vi "TCP - Asynchronous Read of One JSON Message.vi"(8 "error in":errorcluster, 11 "TCP Network Connection in":refnum<k5>) -> (0 "error out":errorcluster, 2 "Received JSON Message":string, 3 "TCP Network Connection out":refnum<k5>)   [LabVIEW 2021]
doc: "Receive a JSON messsage through TCP"
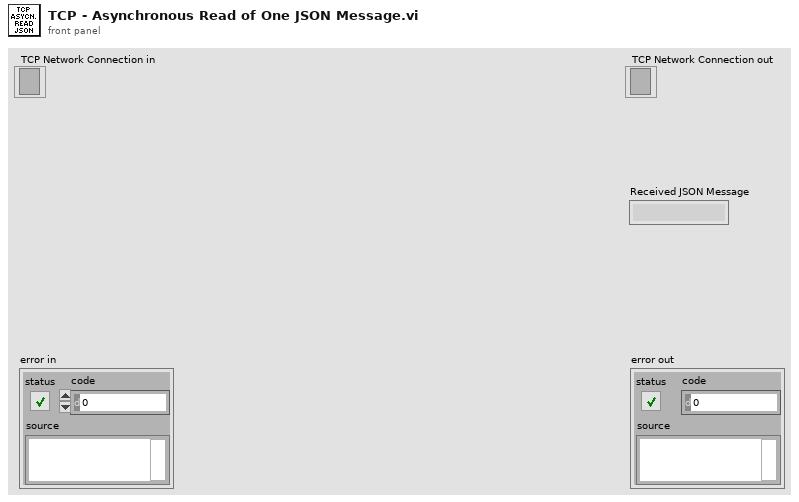
[diagram p1: front panel]
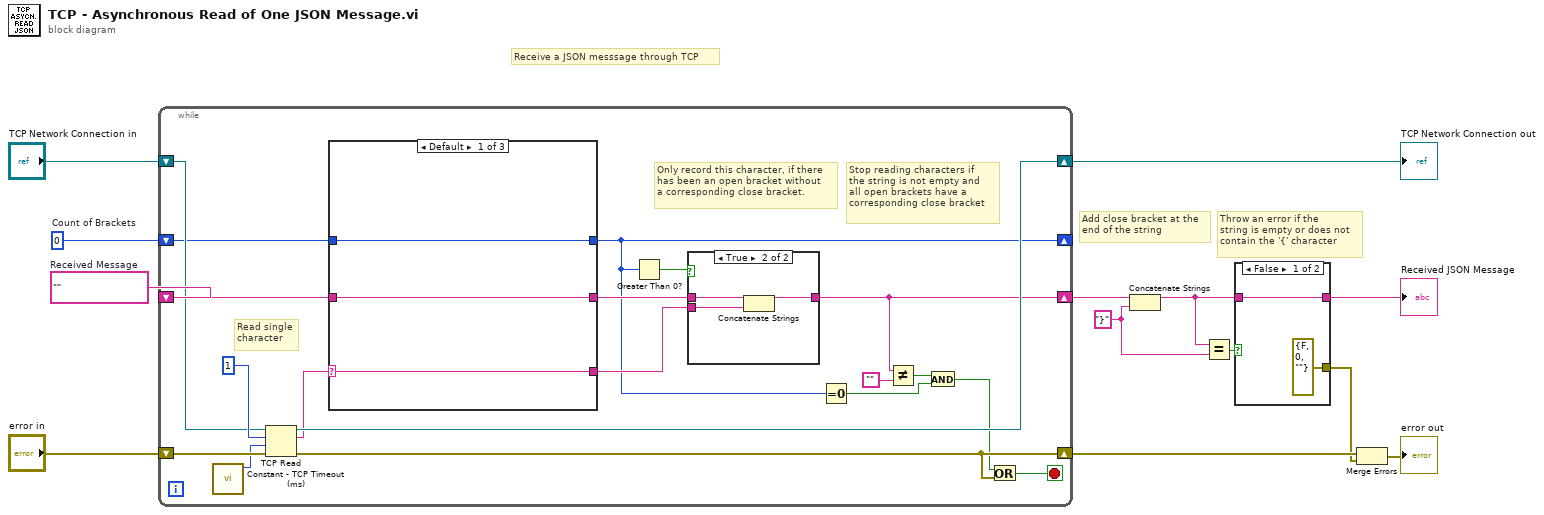
[diagram p0: block diagram]
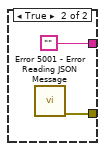
[diagram p2: hidden frame]
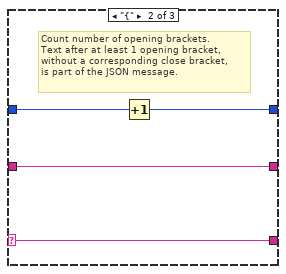
[diagram p4: hidden frame]
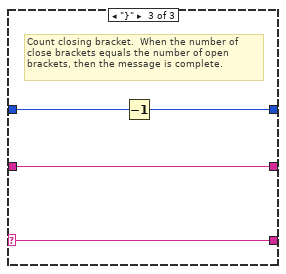
[diagram p5: hidden frame]
diagram:
  w7 = "}" ("string")
  w10 = 0  # Count of Brackets
  w13 = ""  # Received Message
  # "Throw an error if the\nstring is empty or does not\ncontain the '{' character"
  # "Add close bracket at the\nend of the string"
  # "Receive a JSON messsage through TCP"
  n1 = while {
    shift-right: [w27] -> w4
    shift-left: "error in" -> [w32]
    shift-right: [w29] -> w9
    shift-left: "TCP Network Connection in" -> [w30]
    shift-right: [w18] -> w8
    shift-left: w13 -> [w21]
    shift-right: [w17] -> _
    shift-left: w10 -> [w24]
    stop <- w26 stop-if-true
    # "Stop reading characters if\nthe string is not empty and\nall open brackets have a \ncorresponding close bracket"
    # "Only record this character, if there\nhas been an open bracket without\na corresponding close bracket."
    # "Read single\ncharacter"
    n2 = call "Constant - TCP Timeout (ms).vi"() -> ("timeout (ms)"=w28:i32)  [unwired: 11 in]
    n3 = TCP Read(connection ID=w30, bytes to read=1, error in (no error)=w32, 9:w28) -> (connection ID out=w29:refnum<k5>, data out=w25:string, error out=w27:errorcluster)  [unwired: 1 in]
    n4 = case shown="Default" w25 {
      selector: w25 -> [w37 w41 w44]
      tunnel: w24 -> [w39 w43 w47]
      tunnel: [w39 w42 w46] -> w17
      tunnel: [w37 w41 w44] -> w22
      tunnel: w21 -> [w38 w40 w45]
      tunnel: [w38 w40 w45] -> w20
      frame Default {
      }
      frame "{" {
        # "Count number of opening brackets.  \nText after at least 1 opening bracket, \nwithout a corresponding close bracket, \nis part of the JSON message."
        n5 = Increment(x=w43) -> (x+1=w42:i32)
      }
      frame "}" {
        # "Count closing bracket.  When the number of\nclose brackets equals the number of open \nbrackets, then the message is complete."
        n6 = Decrement(x=w47) -> (x-1=w46:i32)
      }
    }
    n7 = Greater Than 0?(x=w17) -> (x > 0?=w23:bool)
    n8 = case shown="True" w23 {
      tunnel: [w33 w36] -> w18
      tunnel: w22 -> [_ w35]
      tunnel: w20 -> [w33 w34]
      frame False {
      }
      frame True {
        n9 = Concatenate Strings(w34, w35) -> (w36:string)
      }
    }
    n10 = Equal To 0?(x=w17) -> (x = 0?=w15:bool)
    n11 = Not Equal?(x=w18, y="") -> (x != y?=w16:bool)
    n12 = And(x=w16, y=w15) -> (x .and. y?=w14:bool)
    n13 = Or(x=w14, y=w27) -> (x .or. y?=w26:bool)
  }
  "TCP Network Connection out" <- w9
  n14 = Concatenate Strings(w8, w7) -> (w1:string)
  n15 = Equal?(x=w1, y=w7) -> (x = y?=w5:bool)
  n16 = case shown="False" w5 {
    tunnel: [errorcluster {"status"=FALSE, "code"=0, "source"=""} ("error out") w51] -> w3
    tunnel: [w48 ""] -> w2
    tunnel: w1 -> [w48 _]
    frame False {
    }
    frame True {
      n17 = call "Error 5001 - Error Reading JSON Message.vi"() -> ("error out"=w51:errorcluster)  [unwired: 11 in]
    }
  }
  "Received JSON Message" <- w2
  n18 = Merge Errors(w4, w3) -> (→"error out":errorcluster)
